vi "Intake Motor Control.vi"(1 "Release Constant":dbl=0.6, 2 "Intake Constant":dbl=-0.6, 3 "Release Button Input":bool, 4 "Intake Button Input":bool) -> (0 "New Scalar":dbl)   [LabVIEW 2019]
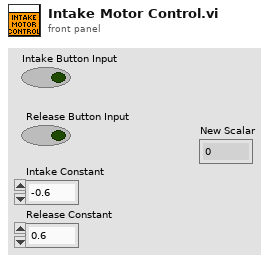
[diagram p1: front panel]
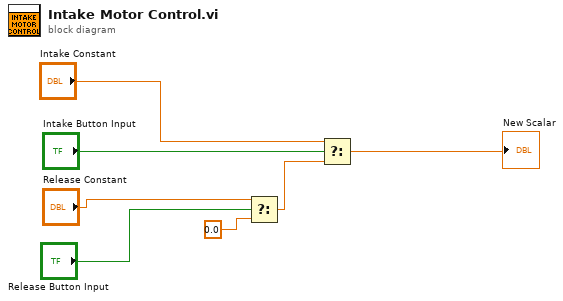
[diagram p0: block diagram]
diagram:
  n1 = Select(t="Release Constant", s="Release Button Input", f=0.0) -> (s? t:f=w6:dbl)
  n2 = Select(t="Intake Constant", s="Intake Button Input", f=w6) -> (s? t:f=→"New Scalar":dbl)
